vi "newDotNetStep.vi"(0 "Engine reference":refnum<k7>, 5 "stepType":string="Action", 7 "Step Name":string, 9 "Requirement":string, 11 "error in":errorcluster, 12 "RecordResult":bool=TRUE, 13 "RecordReq":bool=TRUE) -> (4 "Engine reference(out)":refnum<k7>, 6 "NewStep (out)":refnum<k7>, 8 "dotNetModule(out)":refnum<k7>, 15 "error out":errorcluster)   [LabVIEW 2010]
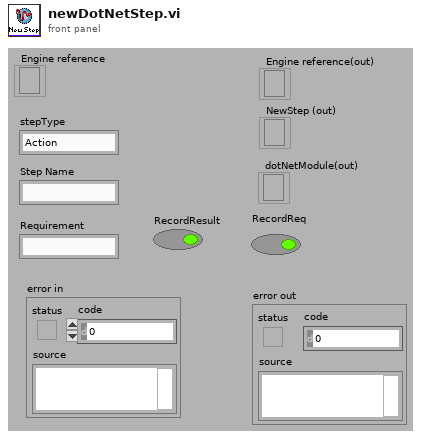
[diagram p1: front panel]
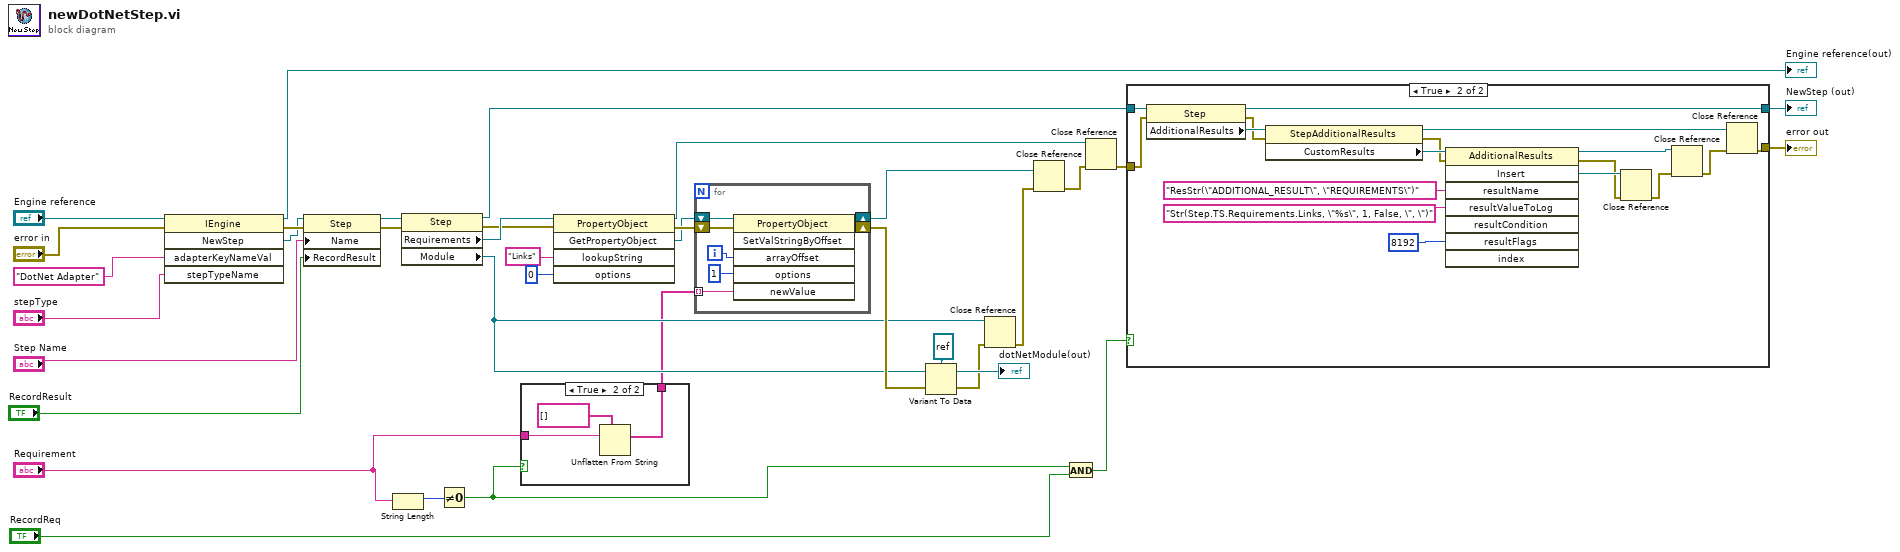
[diagram p0: block diagram]
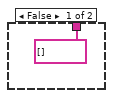
[diagram p2: hidden frame]
diagram:
  n1 = invoke class="IEngine" method="NewStep"(reference="Engine reference", error in="error in", "adapterKeyNameVal"="DotNet Adapter", "stepTypeName"="stepType") -> (reference out=→"Engine reference(out)":refnum<k7>, error out=w30:errorcluster, "NewStep"=w22:refnum<k7>)  [unwired: 1 in, 2 out]
  n2 = property class="Step"(reference=w22, error in=w30, "Name"="Step Name", "RecordResult"="RecordResult") -> (reference out=w11:refnum<k7>, error out=w20:errorcluster)
  n3 = String Length(string="Requirement") -> (length=w5:i32)
  n4 = property class="Step"(reference=w11, error in=w20) -> (reference out=w10:refnum<k7>, error out=w19:errorcluster, "Requirements"=w21:refnum<k7>, "Module"=w14:refnum<k7>)
  n5 = Not Equal To 0?(x=w5) -> (x != 0?=w2:bool)
  n6 = case shown="True" w2 {
    tunnel: "Requirement" -> [_ w40]
    tunnel: [string[] [] w39] -> w1
    frame False {
    }
    frame True {
      n7 = Unflatten From String(type=string[] [], binary string=w40) -> (value=w39:string[])  [unwired: 3 in, 2 out]
    }
  }
  n8 = invoke class="PropertyObject" method="GetPropertyObject"(reference=w21, error in=w19, "lookupString"="Links", "options"=0) -> (reference out=w25:refnum<k7>, error out=w36:errorcluster, "GetPropertyObject"=w35:refnum<k7>)  [unwired: 1 in, 2 out]
  n9 = for {
    tunnel: w1 -> [w41] mode=indexing
    shift-right: [w44] -> w26
    shift-left: w35 -> [w45]
    shift-right: [w43] -> w16
    shift-left: w36 -> [w47]
    i -> [w42]
    n10 = invoke class="PropertyObject" method="SetValStringByOffset"(reference=w45, error in=w47, "arrayOffset"=w42, "options"=1, "newValue"=w41) -> (reference out=w44:refnum<k7>, error out=w43:errorcluster)  [unwired: 1 in, 4 out]
  }
  n11 = Variant To Data(error in=w16, Variant=w14, type=refnum<k7> refnum ("Module")) -> (error out=w15:errorcluster, data=→"dotNetModule(out)":refnum<k7>)
  n12 = Close Reference(reference=w14, error in (no error)=w15) -> (error out=w13:errorcluster)
  n13 = Close Reference(reference=w26, error in (no error)=w13) -> (error out=w24:errorcluster)
  n14 = And(x=w2, y="RecordReq") -> (x .and. y?=w4:bool)
  n15 = Close Reference(reference=w25, error in (no error)=w24) -> (error out=w7:errorcluster)
  n16 = case shown="True" w4 {
    tunnel: w10 -> [w49 w54]
    tunnel: [w49 w53] -> w9
    tunnel: w7 -> [w48 w52]
    tunnel: [w48 w51] -> w8
    frame False {
    }
    frame True {
      n17 = property class="Step"(reference=w54, error in=w52) -> (reference out=w53:refnum<k7>, error out=w50:errorcluster, "AdditionalResults"=w66:refnum<k7>)
      n18 = property class="StepAdditionalResults"(reference=w66, error in=w50) -> (reference out=w58:refnum<k7>, error out=w64:errorcluster, "CustomResults"=w65:refnum<k7>)
      n19 = invoke class="AdditionalResults" method="Insert"(reference=w65, error in=w64, "resultName"="ResStr(\"ADDITIONAL_RESULT\", \"REQUIREMENTS\")", "resultValueToLog"="Str(Step.TS.Requirements.Links, \"%s\", 1, False, \", \")", "resultFlags"=8192) -> (reference out=w60:refnum<k7>, error out=w62:errorcluster, "Insert"=w63:refnum<k7>)  [unwired: 3 in, 5 out]
      n20 = Close Reference(reference=w63, error in (no error)=w62) -> (error out=w61:errorcluster)
      n21 = Close Reference(reference=w60, error in (no error)=w61) -> (error out=w59:errorcluster)
      n22 = Close Reference(reference=w58, error in (no error)=w59) -> (error out=w51:errorcluster)
    }
  }
  "error out" <- w8
  "NewStep (out)" <- w9
